vi "Set_BME_G05p_dymmy.vi"() -> ()   [LabVIEW 2009]
uses:
  BME Beispiele/BME DLL/DelayGenerator.dll
  ChnlWithModulo.ctl
  SignalType.ctl
  BME_G05P1Settings.ctl
panel:
  in  "BME_G05P1 Settings":T1={"GateAB?"=FALSE, "Signal Type"=0, "InputTerminated?"=FALSE, "ClockEnabled?"=FALSE, "InternalClockPeriode(µs)"=0.0, "TriggerLevel"=0.0, "PresetValue"=0, "DivideBy"=0, "Clock Source"=0, "Gate Divider"=1, "PositiveGate?"=FALSE, "InternalTrigger?"=FALSE, "InternalArm?"=FALSE, "SWTrigger?"=FALSE, "RisingEdge?"=FALSE, "StopOnPreset?"=FALSE, "ResetWhenDone?"=FALSE, "TriggerEnabled?"=FALSE} {"Gate Divider" min=1 max=1000000; "Clock Source" items=["Internal Oscillator"=1, "External Trigger"=2, "Trigger & Oscillator"=3]; "Signal Type" items=["TTL"=1, "ECL"=2, "NIM"=3]}
  in  "Chnl B":T3={" Delay (µs)"=0.0, "TriggerModulo"=1, "On? (false)"=FALSE, "PositiveVoltage?(true)"=FALSE, "50OhmTerminated? "=FALSE, "25OhmOutput?"=FALSE} {"TriggerModulo" min=1 max=1000000; "Delay (µs)" min=0.0 max=100000000.0 format="%.5f"}
  in  "Chnl A":T3={" Delay (µs)"=0.0, "TriggerModulo"=1, "On? (false)"=FALSE, "PositiveVoltage?(true)"=FALSE, "50OhmTerminated? "=FALSE, "25OhmOutput?"=FALSE} {"TriggerModulo" min=1 max=1000000; "Delay (µs)" min=0.0 max=100000000.0 format="%.5f"}
  in  "Chnl T":T3={" Delay (µs)"=0.0, "TriggerModulo"=1, "On? (false)"=FALSE, "PositiveVoltage?(true)"=FALSE, "50OhmTerminated? "=FALSE, "25OhmOutput?"=FALSE} {"TriggerModulo" min=1 max=1000000; "Delay (µs)" min=0.0 max=100000000.0 format="%.5f"}
  out "Int Trig Message":string="Max. Rep. Rate = 680kHz\nfor 1ms pulse width"
  out "Int Trig Ref":dbl
  out "Prescaler":u32=1 min=1 max=8
  in  "Pulse Width (ms)":dbl=0.2 min=0.2 max=25.5 format="%#.1f"
  in  "B Triggers per Pulse":u32=1 min=1 max=10000000
  in  "A Triggers per Pulse":u32=1 min=1 max=10000000
  in  "T Triggers per Pulse":u32=1 min=1 max=1000000
  in  "Clock Source":u32(ring) items=["Internal Oscillator", "External Trigger", "Trigger & Oscillator"]
  in  "Internal Arming":bool
  in  "B high current output":bool
  in  "B 50ohm output":bool
  in  "B level":bool
  in  "B activity":bool
  in  "B Extra Delay (ms)":dbl min=0.0 max=100000000.0 format="%.5f"
  in  "A high current output":bool
  in  "A 50ohm output":bool
  in  "A level":bool
  in  "A activity":bool
  in  "A Extra Delay (ms)":dbl min=0.0 max=100000000.0 format="%.5f"
  in  "T high current output":bool
  in  "T 50ohm output":bool
  in  "T level":bool
  in  "T activity":bool
  in  "T Extra Delay (ms)":dbl min=0.0 max=100000000.0 format="%.5f"
  in  "Operation":bool
  in  "Stop on Preset":bool
  in  "Software Trigger":bool
  in  "Positive Gate":bool
  in  "Gate AB":bool
  in  "Clock":bool
  in  "Output":bool
  in  "Slope":bool
  in  "Trigger Source":bool
  in  "Internal Trigger\nRepetition Rate (Hz)":dbl=0.02 min=0.02 max=650000.0 format="%.2f"
  in  "Output Level":u32(ring) items=["TTL", "ECL", "NIM"]
  in  "Gate Divider":i32=1 min=1 max=1000000
  in  "Preset Value":i32 min=0 max=10000000
  in  "External Trigger\nLevel (V)":dbl min=-2.5 max=2.5 format="%.2f"
  in  "Activate":bool
  out "set_BME_05":i32
  in  "Deactivate":bool
  out "output param 21":i32
  out "output param 6":u32
  in  "Stop":bool
  out "output param 20":u32
  out "output param 4":i32
  out "output param 2":i32
  out "DG_Product":i32
  out "Slot Number":i32
  out "Master":i32
  out "DG_Number":i32
  out "output param 1":i32
  out "Number of Cards":i32
  out "p_Error 2":i32
  # "Control of one BME SG02p Delay Generator"
  # "BME Card Information"
  # "Output Channel Settings"
  # "State"
  # "Pulse Sense"
  # "Extra Delay (ms)"
  # "Triggers per Pulse"
  # "50 ohm Output"
  # "25 ohm Output"
  # "T"
  # "A"
  # "B"
  # "Output Settings"
  # "Clock Settings"
  # "Trigger Settings"
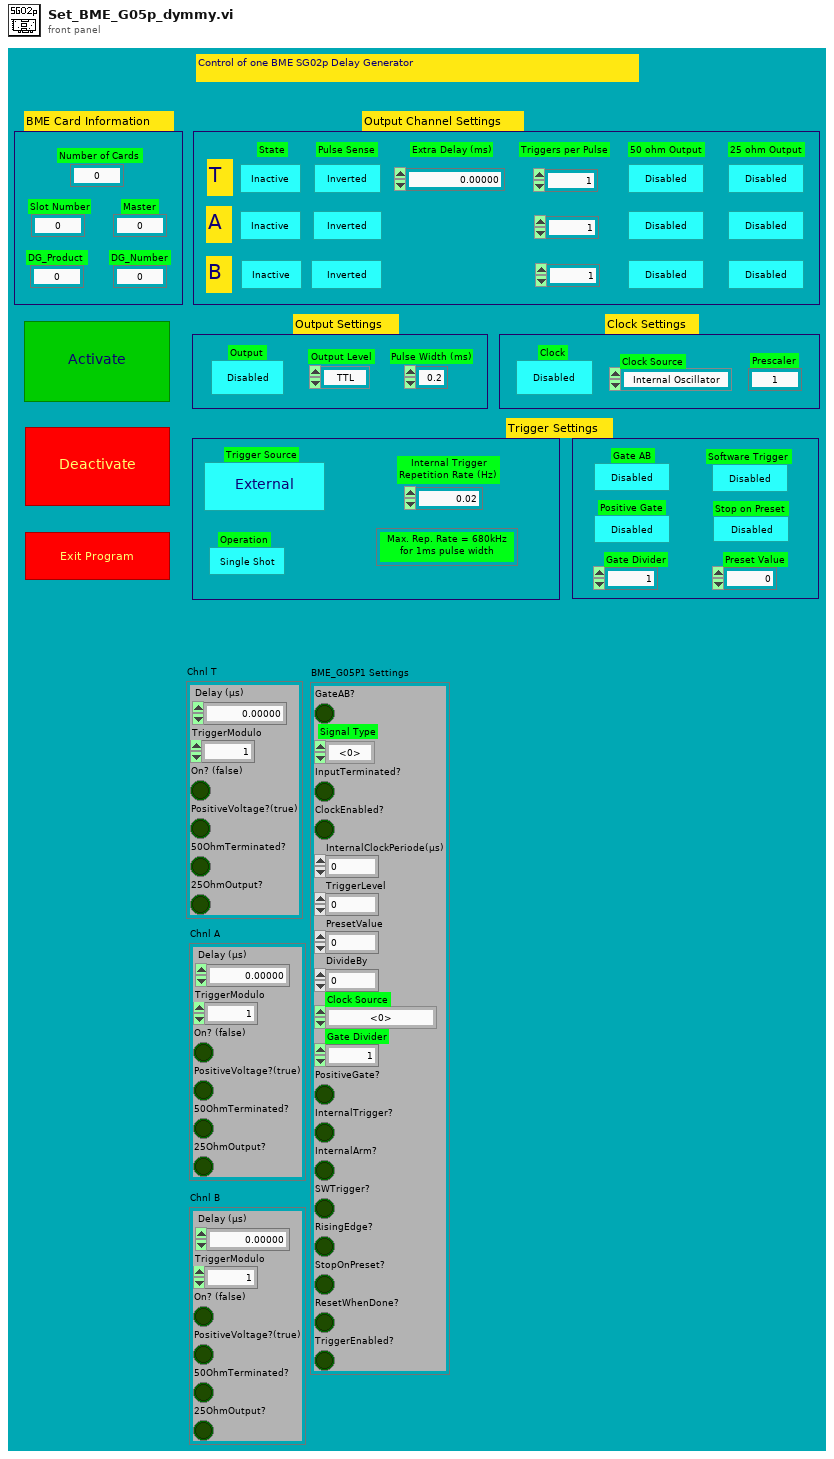
[diagram p1: front panel]
types:
  T1 = typedef "BME_G05P1Settings.ctl" = cluster{"GateAB?":bool, "Signal Type":T2, "InputTerminated?":bool, "ClockEnabled?":bool, "InternalClockPeriode(µs)":dbl, "TriggerLevel":dbl, "PresetValue":i32, "DivideBy":i32, "Clock Source":u32, "Gate Divider":i32, "PositiveGate?":bool, "InternalTrigger?":bool, "InternalArm?":bool, "SWTrigger?":bool, "RisingEdge?":bool, "StopOnPreset?":bool, "ResetWhenDone?":bool, "TriggerEnabled?":bool}
  T2 = typedef "SignalType.ctl" = u32
  T3 = typedef "ChnlWithModulo.ctl" = cluster{" Delay (µs)":dbl, "TriggerModulo":u32, "On? (false)":bool, "PositiveVoltage?(true)":bool, "50OhmTerminated? ":bool, "25OhmOutput?":bool}
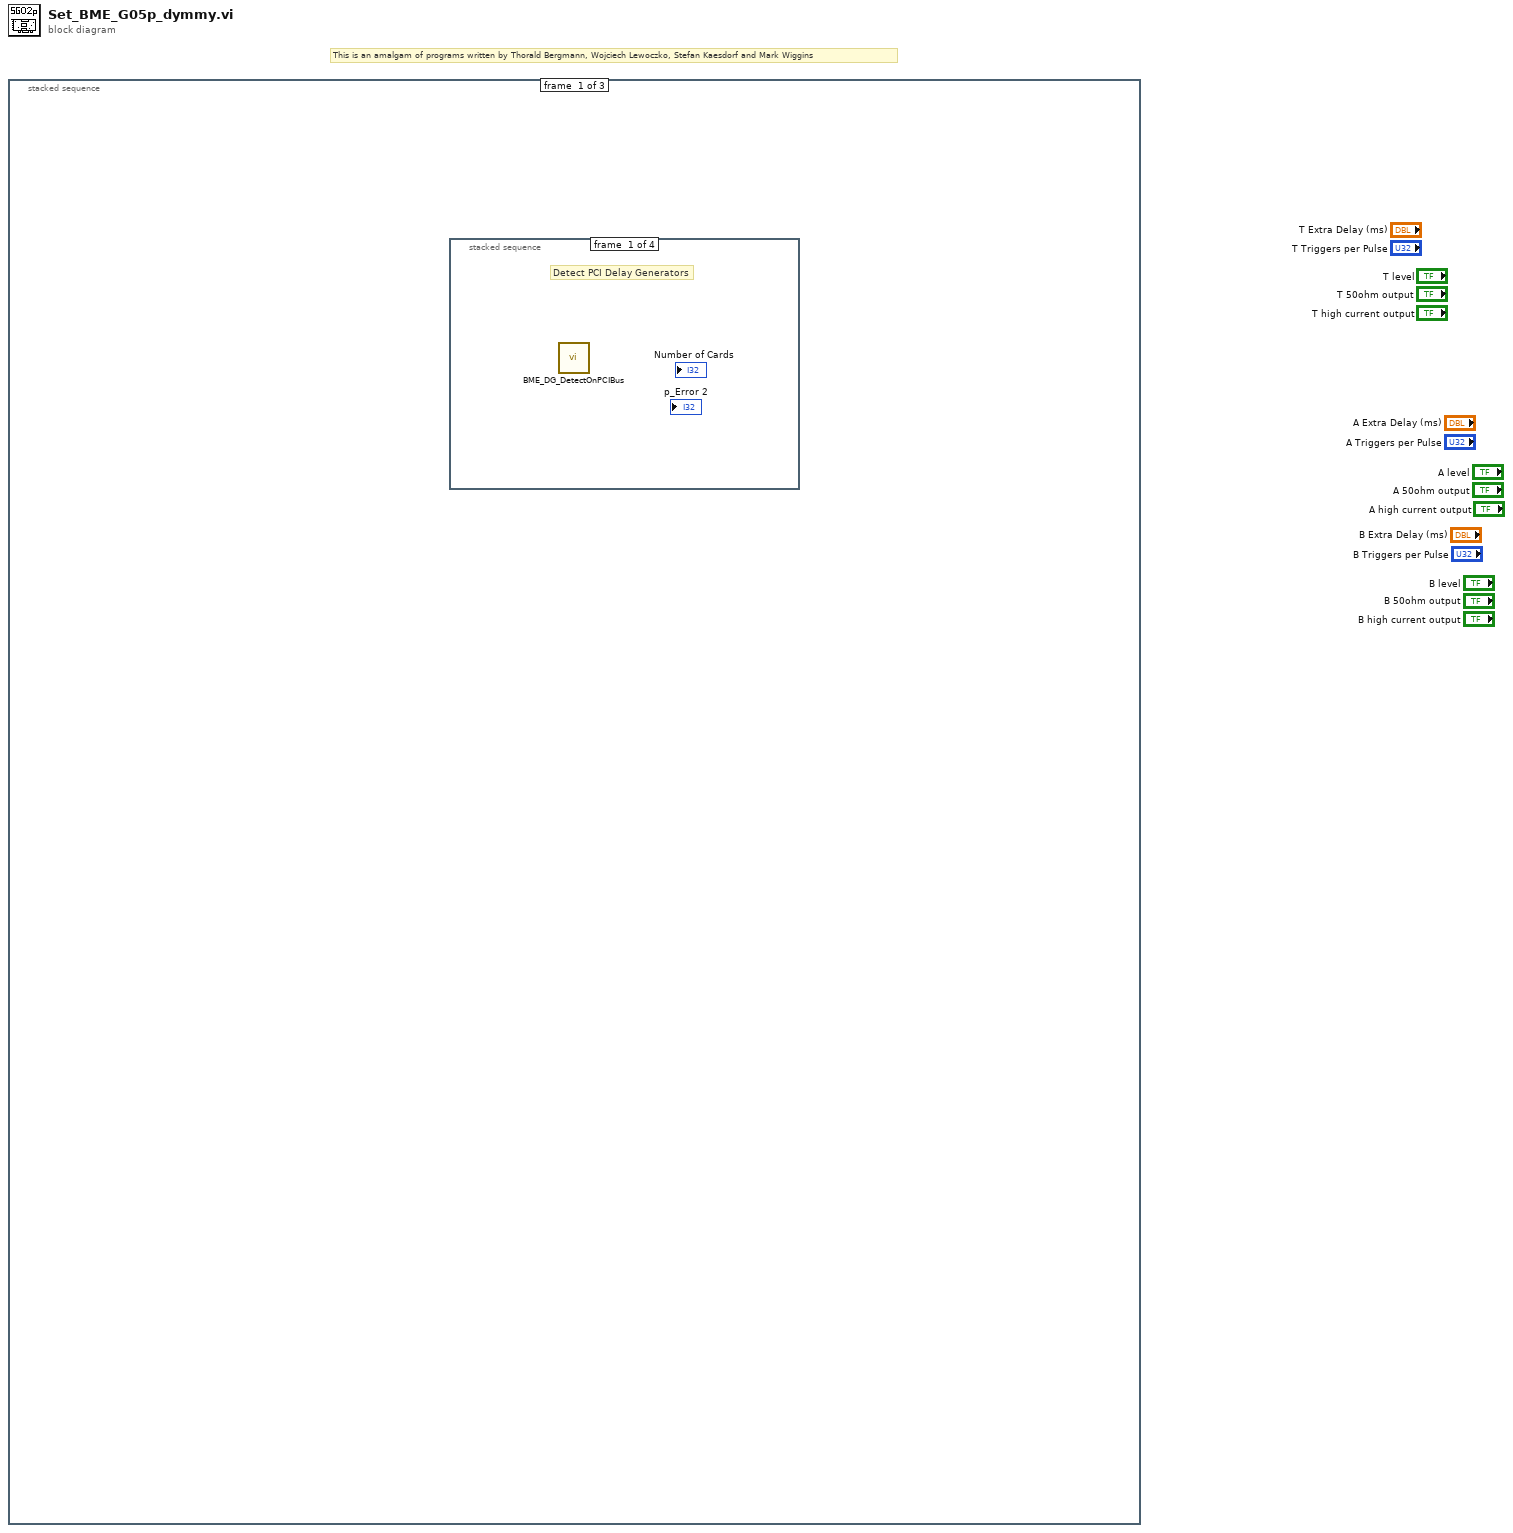
[diagram p0: block diagram]
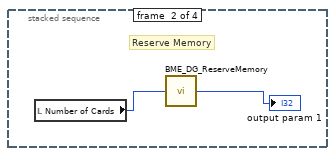
[diagram p2: hidden frame]
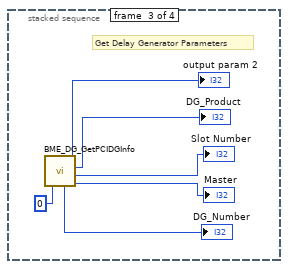
[diagram p3: hidden frame]
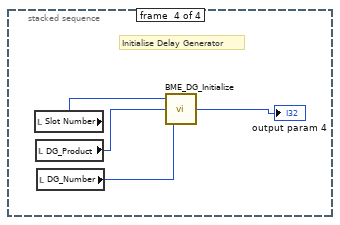
[diagram p4: hidden frame]
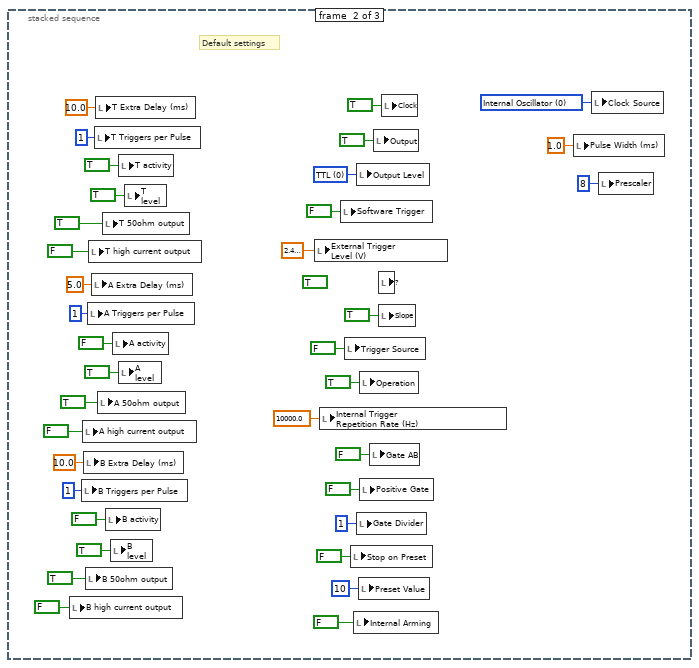
[diagram p5: hidden frame]
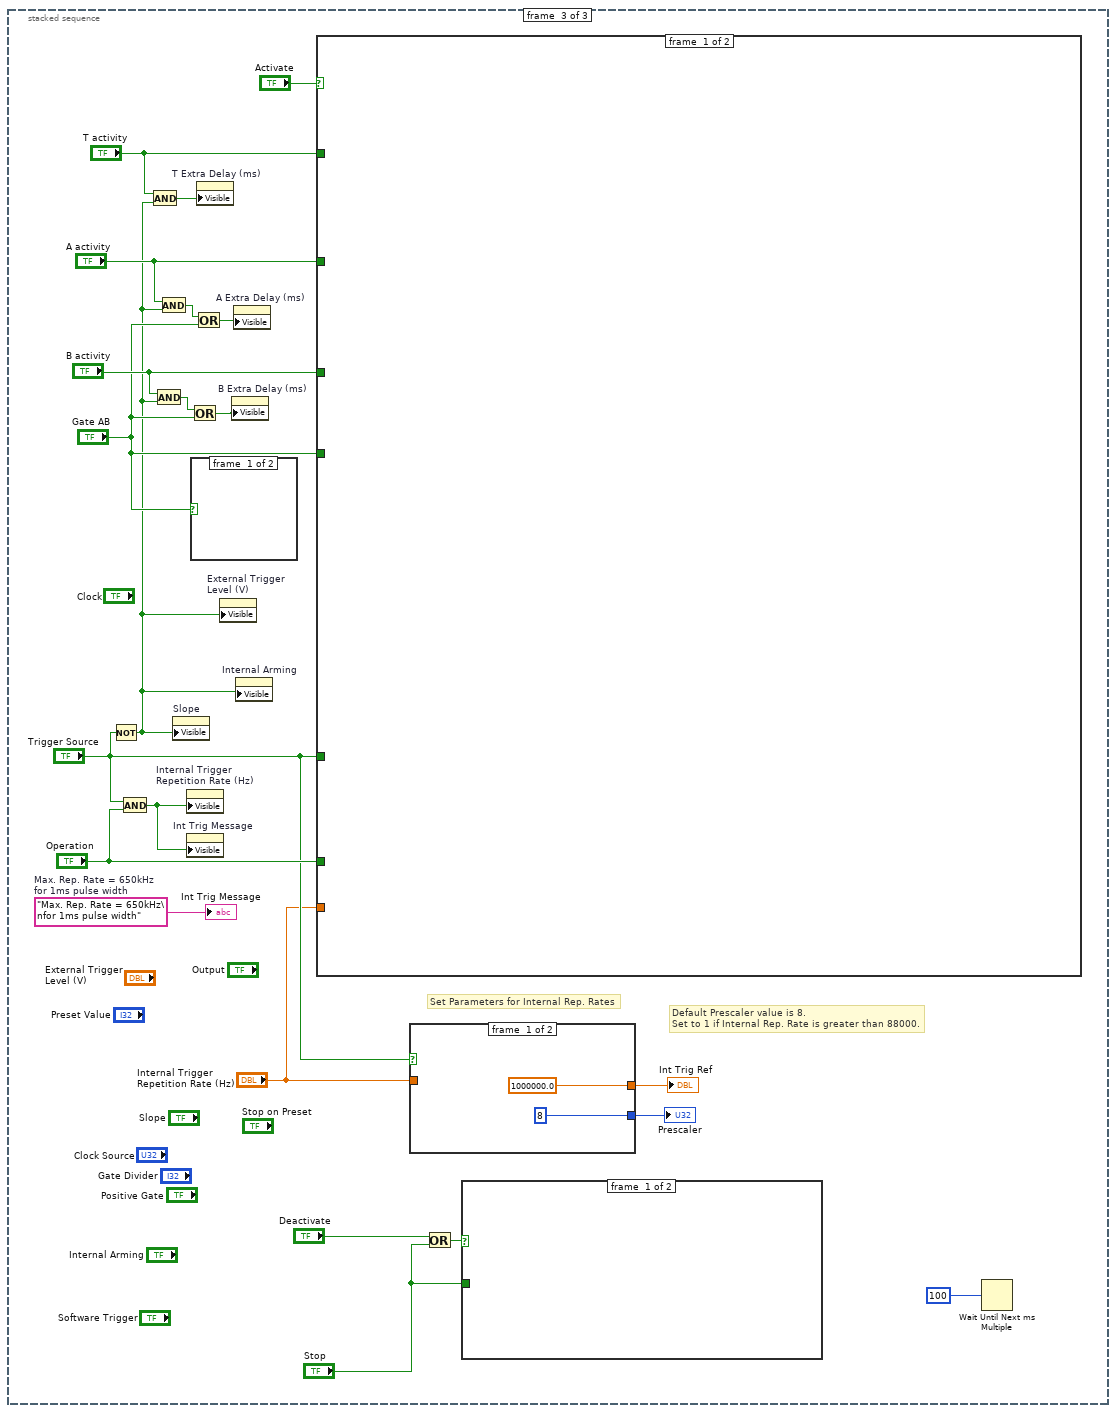
[diagram p6: hidden frame]
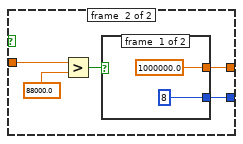
[diagram p7: hidden frame]
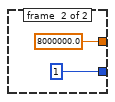
[diagram p8: hidden frame]
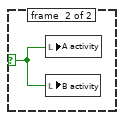
[diagram p9: hidden frame]
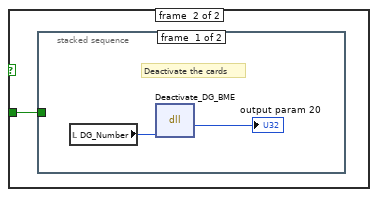
[diagram p10: hidden frame]
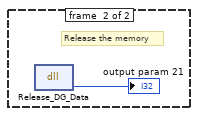
[diagram p12: hidden frame]
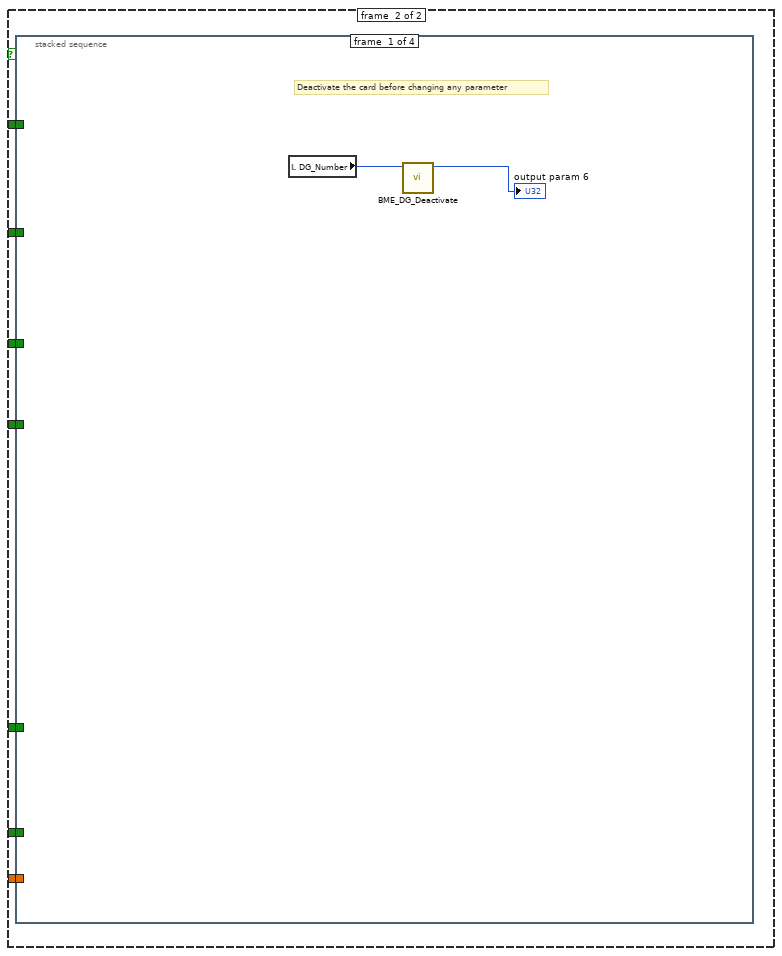
[diagram p13: hidden frame]
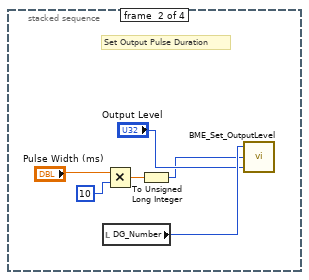
[diagram p14: hidden frame]
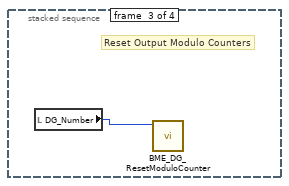
[diagram p15: hidden frame]
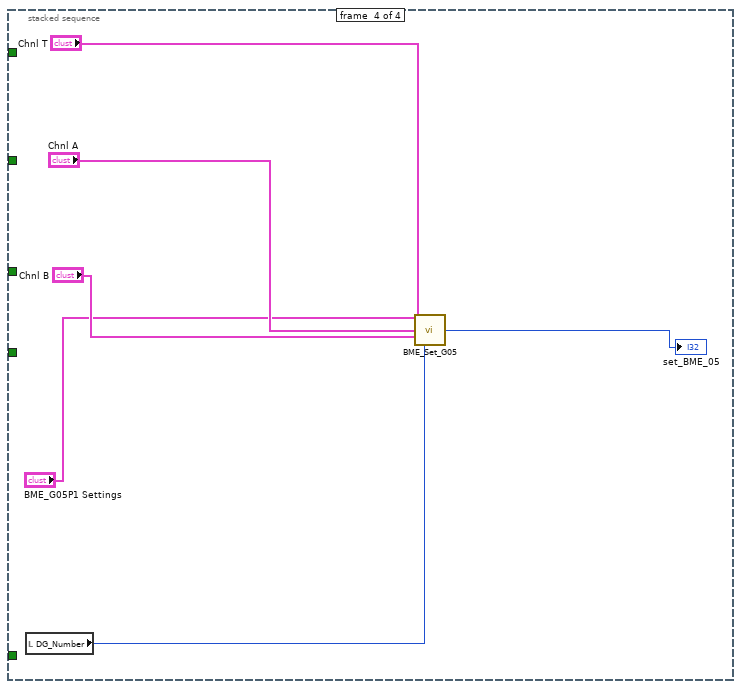
[diagram p16: hidden frame]
diagram:
  # "This is an amalgam of programs written by Thorald Bergmann, Wojciech Lewoczko, Stefan Kaesdorf and Mark Wiggins"
  n1 = stacked-sequence {
    frame #0 {
      n2 = stacked-sequence {
        frame #0 {
          # "Detect PCI Delay Generators"
          n3 = call "BME_DG_DetectOnPCIBus.vi"() -> ()  [unwired: 9 in, 3 out]
        }
        frame #1 {
          # "Reserve Memory"
          n4 = local read "Number of Cards"() -> (w1:i32)
          n5 = call "BME_DG_ReserveMemory.vi"("Number of Cards"=w1) -> ("error code"=→"output param 1":i32)
        }
        frame #2 {
          # "Get Delay Generator Parameters"
          n6 = call "BME_DG_GetPCIDGInfo.vi"("DG_Number 2"=0 ("DG_Number")) -> ("Master"=→"Master":i32, "SlotNumber"=→"Slot Number":i32, "DG_Product"=→"DG_Product":i32, "Numeric"=→"output param 2":i32, "DG_Number"=→"DG_Number":i32)
        }
        frame #3 {
          # "Initialise Delay Generator"
          n7 = local read "Slot Number"() -> (w10:i32)
          n8 = local read "DG_Product"() -> (w11:i32)
          n9 = local read "DG_Number"() -> (w12:i32)
          n10 = call "BME_DG_Initialize.vi"("DG_Number"=w12, "DG_Product"=w11, "Slot Number"=w10) -> ("Numeric"=→"output param 4":i32)
        }
      }
    }
    frame #1 {
      w15 = u32 0 items=["Internal Oscillator", "External Trigger", "Trigger & Oscillator"] ("Clock Source")
      (unwired) TRUE ("Input Impendance")
      w43 = u32 0 items=["TTL", "ECL", "NIM"] ("Output Level")
      # "Default settings"
      n11 = local write "B high current output"(FALSE ("B higher terms")) -> ()
      n12 = local write "B Triggers per Pulse"(u32 1 ("Tb_output_modulo")) -> ()
      n13 = local write "A high current output"(FALSE ("A higher terms")) -> ()
      n14 = local write "B Extra Delay (ms)"(10.0 ("B Extra Delay (us)")) -> ()
      n15 = local write "B 50ohm output"(TRUE ("B base term")) -> ()
      n16 = local write "A Triggers per Pulse"(u32 1 ("Ta_output_modulo")) -> ()
      n17 = local write "T high current output"(FALSE ("T higher terms")) -> ()
      n18 = local write "A Extra Delay (ms)"(5.0 ("A Extra Delay (us)")) -> ()
      n19 = local write "T Triggers per Pulse"(u32 1 ("T0_output_modulo")) -> ()
      n20 = local write "T Extra Delay (ms)"(10.0 ("T Extra Delay (us)")) -> ()
      n21 = local write "A 50ohm output"(TRUE ("A base term")) -> ()
      n22 = local write "T 50ohm output"(TRUE ("T base term")) -> ()
      n23 = local write "B activity"(FALSE ("B activity")) -> ()
      n24 = local write "B level"(TRUE ("B level")) -> ()
      n25 = local write "A activity"(FALSE ("A activity")) -> ()
      n26 = local write "T activity"(TRUE ("T activity")) -> ()
      n27 = local write "A level"(TRUE ("A level")) -> ()
      n28 = local write "T level"(TRUE ("T level")) -> ()
      n29 = local write "External Trigger\nLevel (V)"(2.4999999999999982 ("External Trigger\nLevel (V)")) -> ()
      n30 = local write "Internal Trigger\nRepetition Rate (Hz)"(10000.0 ("Internal Trigger\nRepetition Rate (Hz)")) -> ()
      n31 = local write "Software Trigger"(FALSE ("Software Trigger")) -> ()
      n32 = local write "Trigger Source"(FALSE ("Trigger Source")) -> ()
      n33 = local write "Stop on Preset"(FALSE ("Stop on Preset")) -> ()
      n34 = local write "Internal Arming"(FALSE ("IntArm")) -> ()
      n35 = local write "Output Level"(w43) -> ()
      n36 = local write "Gate Divider"(1 ("Gate Divider")) -> ()
      n37 = local write "Preset Value"(10 ("Preset Value")) -> ()
      n38 = local write "Operation"(TRUE ("Operation")) -> ()
      n39 = local write "Positive Gate"(FALSE ("Positive Gate")) -> ()
      n40 = local write "Gate AB"(FALSE ("Gate AB")) -> ()
      n41 = local write "Output"(TRUE ("Output")) -> ()
      n42 = local read item#-1() -> ()  [unwired: 1 in]
      n43 = local write "Slope"(TRUE ("Slope")) -> ()
      n44 = local write "Clock"(TRUE ("Clock")) -> ()
      n45 = local write "Pulse Width (ms)"(1.0 ("Pulse Width (ms)")) -> ()
      n46 = local write "Clock Source"(w15) -> ()
      n47 = local write "Prescaler"(u32 8 ("Prescaler")) -> ()
    }
    frame #2 {
      w50 = "Max. Rep. Rate = 650kHz\nfor 1ms pulse width"  # Max. Rep. Rate = 650kHz for 1ms pulse width
      # "Default Prescaler value is 8.\nSet to 1 if Internal Rep. Rate is greater than 88000."
      # "Set Parameters for Internal Rep. Rates"
      n48 = Not(x="Trigger Source") -> (.not. x?=w55:bool)
      n49 = And(x="Trigger Source", y="Operation") -> (x .and. y?=w49:bool)
      n50 = And(x="T activity", y=w55) -> (x .and. y?=w65:bool)
      n51 = And(x="B activity", y=w55) -> (x .and. y?=w57:bool)
      n52 = And(x="A activity", y=w55) -> (x .and. y?=w60:bool)
      n53 = property on="Slope" class="Boolean (strict)"("Visible"=w55) -> ()  [unwired: 2 in, 2 out]
      n54 = property on="Internal Trigger\nRepetition Rate (Hz)" class="Digital (strict)"("Visible"=w49) -> ()  [unwired: 2 in, 2 out]
      n55 = property on="Int Trig Message" class="String"("Visible"=w49) -> ()  [unwired: 2 in, 2 out]
      n56 = Or(x=w57, y="Gate AB") -> (x .or. y?=w58:bool)
      n57 = case shown="True" "Gate AB" {
        selector: "Gate AB" -> [_ w82]
        frame #0 {
        }
        frame #1 {
          n58 = local write "A activity"(w82) -> ()
          n59 = local write "B activity"(w82) -> ()
        }
      }
      n60 = Or(x=w60, y="Gate AB") -> (x .or. y?=w59:bool)
      n61 = property on="T Extra Delay (ms)" class="Digital (strict)"("Visible"=w65) -> ()  [unwired: 2 in, 2 out]
      n62 = property on="External Trigger\nLevel (V)" class="Digital (strict)"("Visible"=w55) -> ()  [unwired: 2 in, 2 out]
      n63 = property on="B Extra Delay (ms)" class="Digital (strict)"("Visible"=w58) -> ()  [unwired: 2 in, 2 out]
      n64 = property on="A Extra Delay (ms)" class="Digital (strict)"("Visible"=w59) -> ()  [unwired: 2 in, 2 out]
      n65 = property on="Internal Arming" class="Boolean (strict)"("Visible"=w55) -> ()  [unwired: 2 in, 2 out]
      n66 = case shown="True" "Activate" {
        tunnel: "Trigger Source" -> [_ w89]
        tunnel: "Operation" -> [_ w94]
        tunnel: "T activity" -> [_ w93]
        tunnel: "A activity" -> [_ w92]
        tunnel: "B activity" -> [_ w91]
        tunnel: "Gate AB" -> [_ w90]
        tunnel: "Internal Trigger\nRepetition Rate (Hz)" -> [_ w88]
        frame #0 {
        }
        frame #1 {
          n67 = stacked-sequence {
            tunnel: w94 -> [_ _ _ _]
            tunnel: w93 -> [_ _ _ _]
            tunnel: w92 -> [_ _ _ _]
            tunnel: w91 -> [_ _ _ _]
            tunnel: w90 -> [_ _ _ _]
            tunnel: w89 -> [_ _ _ _]
            tunnel: w88 -> [_ _ _ _]
            frame #0 {
              # "Deactivate the card before changing any parameter"
              n68 = local read "DG_Number"() -> (w95:i32)
              n69 = call "BME_DG_Deactivate.vi"("DG_Number"=w95) -> ("return value"=→"output param 6":u32)  [unwired: 9 in, 1 out]
            }
            frame #1 {
              # "Set Output Pulse Duration"
              n70 = local read "DG_Number"() -> (w102:i32)
              n71 = Multiply(x="Pulse Width (ms)", y=u32 10) -> (x*y=w98:dbl)
              n72 = To Unsigned Long Integer(number=w98) -> (unsigned 32bit integer=w97:u32)
              n73 = call "BME_Set_OutputLevel.vi"("Output Level"="Output Level", "Numeric"=w97, "DG_Number"=w102) -> ()
            }
            frame #2 {
              # "Reset Output Modulo Counters"
              n74 = local read "DG_Number"() -> (w103:i32)
              n75 = call "BME_DG_ResetModuloCounter.vi"("DG_Number"=w103) -> ()  [unwired: 10 in, 1 out]
            }
            frame #3 {
              n76 = local read "DG_Number"() -> (w109:i32)
              n77 = call "BME_Set_G05.vi"("BME_G05P1 Settings"="BME_G05P1 Settings", "DG_Number"=w109, "Chnl T"="Chnl T", "Chnl A"="Chnl A", "Chnl B"="Chnl B") -> ("return value"=→"set_BME_05":i32)  [unwired: 9 in, 1 out]
            }
          }
        }
      }
      n78 = case shown="True" "Trigger Source" {
        tunnel: "Internal Trigger\nRepetition Rate (Hz)" -> [_ w74]
        tunnel: [8 w75] -> w54
        tunnel: [1000000.0 ("Int Trig Ref") w73] -> w52
        frame #0 {
        }
        frame #1 {
          n79 = Greater?(x=w74, y=88000.0) -> (0:w76:bool)
          n80 = case shown="True" w76 {
            tunnel: [8 1] -> w75
            tunnel: [1000000.0 ("Int Trig Ref") 8000000.0 ("Int Trig Ref")] -> w73
            frame #0 {
            }
            frame #1 {
            }
          }
        }
      }
      "Prescaler" <- w54
      "Int Trig Ref" <- w52
      n81 = Or(x="Deactivate", y="Stop") -> (x .or. y?=w69:bool)
      n82 = case shown="True" w69 {
        tunnel: "Stop" -> [_ w83]
        frame #0 {
        }
        frame #1 {
          n83 = stacked-sequence {
            tunnel: w83 -> [_ w86]
            frame #0 {
              # "Deactivate the cards"
              n84 = local read "DG_Number"() -> (w84:i32)
              n85 = dll-call lib="C:/Dokumente und Einstellungen/A2.5/Desktop/BME Beispiele/BME DLL/DelayGenerator.dll" fn="Deactivate_DG_BME"("DG_Number"=w84) -> (→"output param 20":u32)  [unwired: 4 in, 2 out]
            }
            frame #1 {
              n86 = case shown="True" w86 {
                frame #0 {
                }
                frame #1 {
                  # "Release the memory"
                  n87 = dll-call lib="C:/Dokumente und Einstellungen/A2.5/Desktop/BME Beispiele/BME DLL/DelayGenerator.dll" fn="Release_DG_Data"() -> (→"output param 21":i32)  [unwired: 3 in, 2 out]
                }
              }
            }
          }
        }
      }
      n88 = Wait Until Next ms Multiple(millisecond multiple=u32 100) -> ()  [unwired: 1 out]
      "Int Trig Message" <- w50
    }
  }
